vi "Read Sizing.vi"(11 "Flex Subpanel in":refnum<class "Flex UI Subpanel.lvclass">) -> (2 "Sizing":T1, 3 "Flex Subpanel out":refnum<class "Flex UI Subpanel.lvclass">)   [LabVIEW 2016, in "Flex UI Subpanel.lvclass"]
uses:
  Flex UI Subpanel.lvclass
  Enum - Sizing.ctl
  Flex UI Subpanel.lvclass/Flex UI Subpanel.ctl
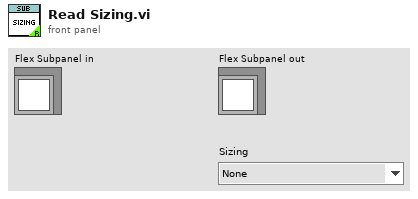
[diagram p1: front panel]
types:
  T1 = typedef "Flex UI Subpanel.lvclass/Enum - Sizing.ctl" = enum16{"None", "Largest Decoration", "Maximize"}
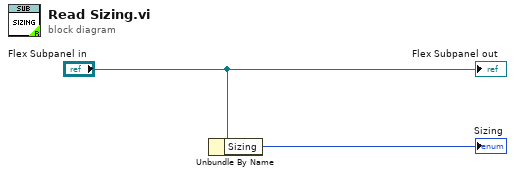
[diagram p0: block diagram]
diagram:
  n1 = Unbundle By Name("Flex Subpanel in") -> ("Sizing"=→"Sizing":T1)
  "Flex Subpanel out" <- "Flex Subpanel in"
